vi "context.vi"(8 "error in (no error)":errorcluster, 11 "Context in":refnum<class "Context.lvclass">) -> (0 "error out":errorcluster, 3 "Context out":refnum<class "Context.lvclass">)   [LabVIEW 2018, in "Context.lvclass"]
doc: "This is a constructor VI, which builds, configures and returns a context to the calling code."
uses:
  Context.lvclass
  Initialize/Initialize.lvclass
  C:/Users/fflores/Documents/OOP-State-Machine/State/State.lvclass
  ContextData/ContextData.lvclass
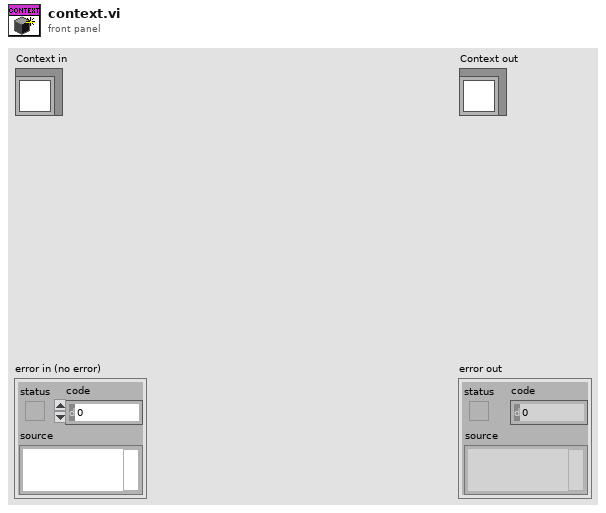
[diagram p1: front panel]
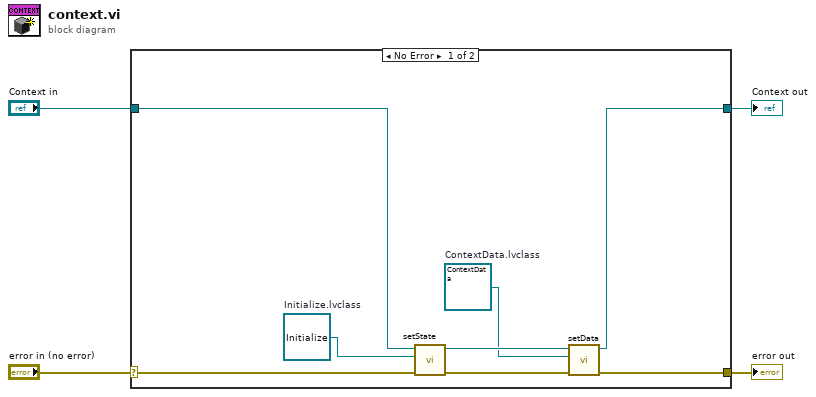
[diagram p0: block diagram]
diagram:
  n1 = case shown="No Error" "error in (no error)" {
    selector: "error in (no error)" -> [w12 w14]
    tunnel: [w8 w14] -> w3
    tunnel: [w6 w13] -> w1
    tunnel: "Context in" -> [w10 w13]
    frame No Error {
      w5 = refnum<class "ContextData.lvclass"> refnum  # ContextData.lvclass
      w9 = refnum<class "Initialize.lvclass"> refnum  # Initialize.lvclass
      n2 = call "setState.vi"("error in (no error)"=w12, "State.lvclass"=w9, "Context in"=w10) -> ("error out"=w11:errorcluster, "Context out"=w7:refnum<class "Context.lvclass">)  [unwired: 7 in]
      n3 = call "setData.vi"("error in (no error)"=w11, "ContextData.lvclass"=w5, "Context in"=w7) -> ("error out"=w8:errorcluster, "Context out"=w6:refnum<class "Context.lvclass">)  [unwired: 7 in]
    }
    frame Error {
    }
  }
  "error out" <- w3
  "Context out" <- w1
